vi "Caller Closed.vi"(8 "error in (no error)":errorcluster, 11 "ExecAnchor in":refnum<class "ExecAnchor.lvclass">) -> (0 "error out":errorcluster, 3 "ExecAnchor out":refnum<class "ExecAnchor.lvclass">)   [LabVIEW 2020, in "ExecAnchor.lvclass"]
uses:
  ExecAnchor.lvclass
  ExecAnchor.lvclass/ExecAnchor.ctl
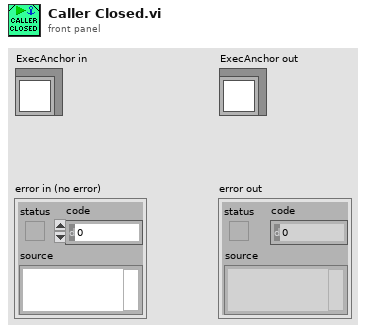
[diagram p1: front panel]
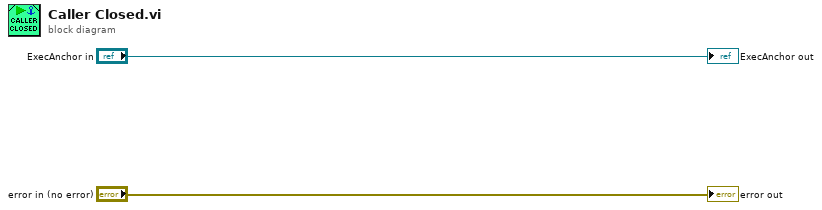
[diagram p0: block diagram]
diagram:
  "error out" <- "error in (no error)"
  "ExecAnchor out" <- "ExecAnchor in"
